vi "read actual temperatures.vi"(7 "Serial Port":refnum<visa-resource-name>) -> (1 "?":T2 {"Flow B" format="%.2f"; "Flow A" format="%.2f"; "Inj B" format="%.2f"; "Det B" format="%.2f"; "Det A" format="%.2f"; "Inj A" format="%.2f"; "Oven" format="%.2f"}, 2 "?":T1 {"Inj B" format="%.2f"; "Det B" format="%.2f"; "Det A" format="%.2f"; "Inj A" format="%.2f"; "Oven" format="%.2f"}, 3 "Serial Port":refnum<visa-resource-name>)   [LabVIEW 2012]
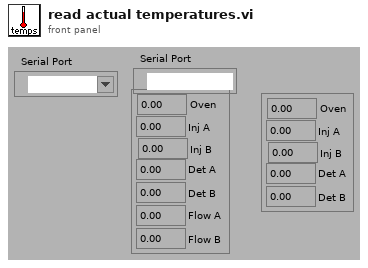
[diagram p1: front panel]
types:
  T1 = cluster{"Oven":dbl, "Inj A":dbl, "Inj B":dbl, "Det A":dbl, "Det B":dbl}
  T2 = cluster{"Oven":dbl, "Inj A":dbl, "Inj B":dbl, "Det A":dbl, "Det B":dbl, "Flow A":dbl, "Flow B":dbl}
  T3 = cluster{"[0]":dbl, "[1]":dbl, "[2]":dbl, "[3]":dbl, "[4]":dbl, "[5]":dbl, "[6]":dbl}
  T4 = cluster{"[0]":dbl, "[1]":dbl, "[2]":dbl, "[3]":dbl, "[4]":dbl}
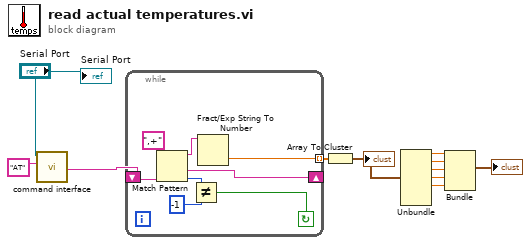
[diagram p0: block diagram]
diagram:
  n1 = call "command interface.vi"("command"="AT", "Serial Port"="Serial Port") -> ("response"=w8:string)  [unwired: 5 in, 3 out]
  n2 = while {
    tunnel: [w16] -> w11 mode=indexing
    shift-left: w8 -> [w19]
    shift-right: [w17] -> _
    stop <- w14 continue-if-true
    n3 = Match Pattern(string=w19, regular expression=",+") -> (before substring=w12:string, after substring=w17:string, offset past match=w15:i32)  [unwired: 1 in, 1 out]
    n4 = Not Equal?(x=w15, y=-1) -> (x != y?=w14:bool)
    n5 = Fract/Exp String To Number(string=w12) -> (number=w16:dbl)  [unwired: 3 in, 1 out]
  }
  n6 = Array To Cluster(array=w11) -> (cluster=w7:T3)
  "?" <- w7
  n7 = Unbundle(w7) -> ("[0]"=w6:dbl, "[1]"=w5:dbl, "[2]"=w4:dbl, "[3]"=w3:dbl, "[4]"=w2:dbl)  [unwired: 2 out]
  n8 = Bundle("[0]"=w6, "[1]"=w5, "[2]"=w4, "[3]"=w3, "[4]"=w2) -> (→"?":T4)  [unwired: 1 in]
  "Serial Port" <- "Serial Port"
